vi "Folder_Create.vi"(8 "Folder Name":string, 11 "Folder Path":string) -> (3 "created path":path)   [LabVIEW 2019]
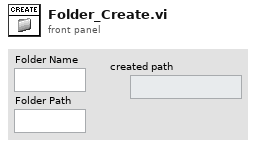
[diagram p1: front panel]
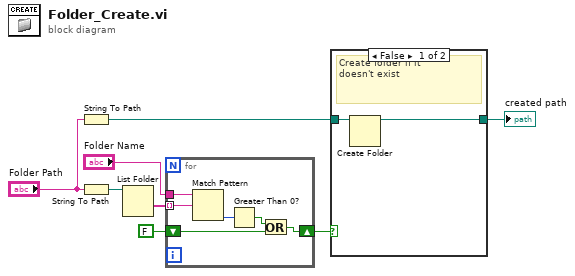
[diagram p0: block diagram]
diagram:
  n1 = String To Path(string="Folder Path") -> (path=w5:path)
  n2 = String To Path(string="Folder Path") -> (path=w2:path)
  n3 = List Folder(path=w2) -> (folder names=w8:string[])  [unwired: 3 in, 3 out]
  n4 = for {
    tunnel: w8 -> [w10] mode=indexing
    tunnel: "Folder Name" -> [w9]
    shift-right: [w12] -> w6
    shift-left: FALSE -> [w11]
    n5 = Match Pattern(string=w9, regular expression=w10) -> (offset past match=w14:i32)  [unwired: 1 in, 3 out]
    n6 = Greater Than 0?(x=w14) -> (x > 0?=w13:bool)
    n7 = Or(x=w13, y=w11) -> (x .or. y?=w12:bool)
  }
  n8 = case shown="False" w6 {
    tunnel: w5 -> [w16 w17]
    tunnel: [w15 w17] -> w3
    frame False {
      # "Create folder if it \ndoesn't exist"
      n9 = Create Folder(path (use dialog)=w16) -> (created path=w15:path)  [unwired: 2 in, 2 out]
    }
    frame True {
    }
  }
  "created path" <- w3
